vi "test distributeControlsEvenly.vi"() -> ()   [LabVIEW 2017]
uses:
  user.lib/_NEVSTOP/Communicable State Machine(CSM)/_tool/_ui/csm-ui-support.lvlib
panel:
  out "String":string
  in  "Numeric 2":dbl
  in  "Numeric":dbl
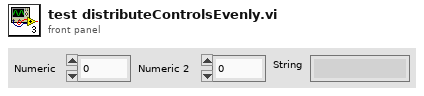
[diagram p1: front panel]
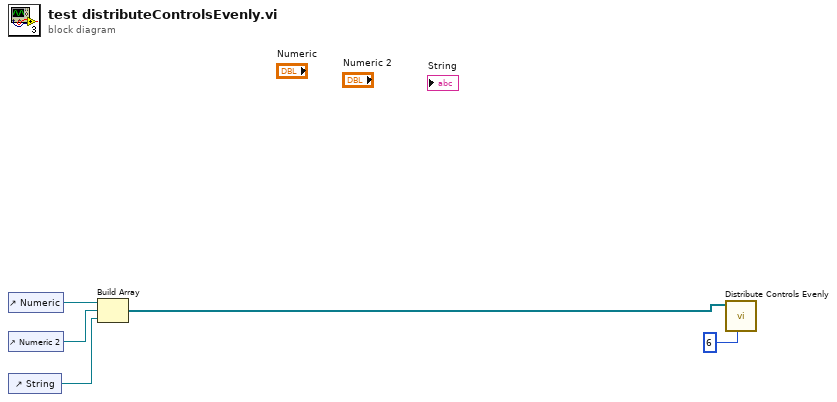
[diagram p0: block diagram]
diagram:
  n1 = control-ref of="Numeric"() -> (w5:refnum<vi>)
  n2 = control-ref of="Numeric 2"() -> (w4:refnum<vi>)
  n3 = control-ref of="String"() -> (w3:refnum<vi>)
  n4 = Build Array(w5, w4, w3) -> (w2:refnum<vi>[])
  n5 = call "Distribute Controls Evenly.vi"("space(6)"=u32 6 ("space(12)"), "Controls"=w2) -> ()  [unwired: 9 in, 1 out]
